vi "Test_Main.vi"   [LabVIEW 2023]
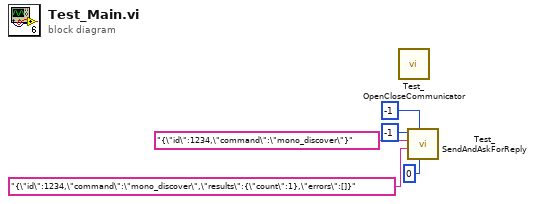
[diagram p0: block diagram]
diagram:
  n1 = call "Test_OpenCloseCommunicator.vi"() -> ()  [unwired: 10 in, 2 out]
  n2 = call "Test_SendAndAskForReply.vi"("Delay between send and receive [ms]"=u32 0, "timeout for receiving data [ms]"=-1, "control answer from\nwebsocket server"="{\"id\":1234,\"command\":\"mono_discover\",\"results\":{\"count\":1},\"errors\":[]}" ("test answer from\nwebsocket server"), "send command"="{\"id\":1234,\"command\":\"mono_discover\"}", "timeout for sending data [ms]"=-1) -> ()  [unwired: 6 in, 1 out]
